vi "ADFGVX.vi"() -> ()   [LabVIEW 2013]
uses:
  <vilib>/Utility/miscctls.llb/LVRowAndColumnTypeDef.ctl
panel:
  out "Intermediate4":string[][](array[string])
  out "Sorted String":string[](array[string])
  out "Intermediate3":string[][](array[string])
  out "Output":string
  out "Intermediate2":string[][](array[string])
  in  "Decrypt":bool
  in  "Encrypt":bool
  in  "Input":string
  out "String1":string caption="Intermediate1"
  in  "String":string
  in  "Stop":bool
  in  "Generate":bool
  in  "Cipher Table":string[][](table)
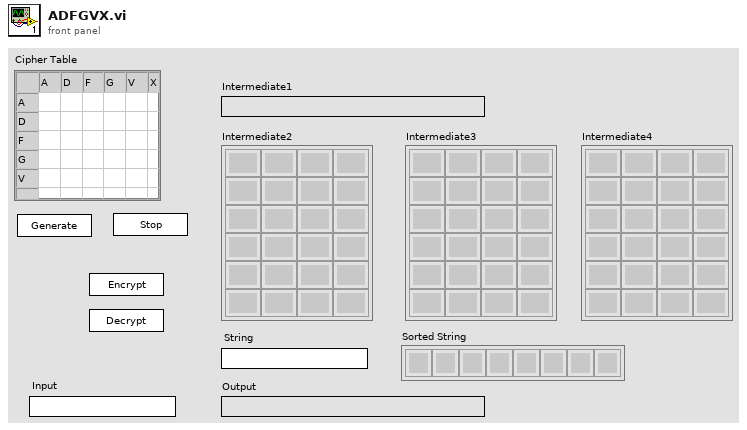
[diagram p1: front panel]
types:
  T1 = typedef "LVRowAndColumnTypeDef.ctl" = cluster{"Row":i32, "Column":i32}
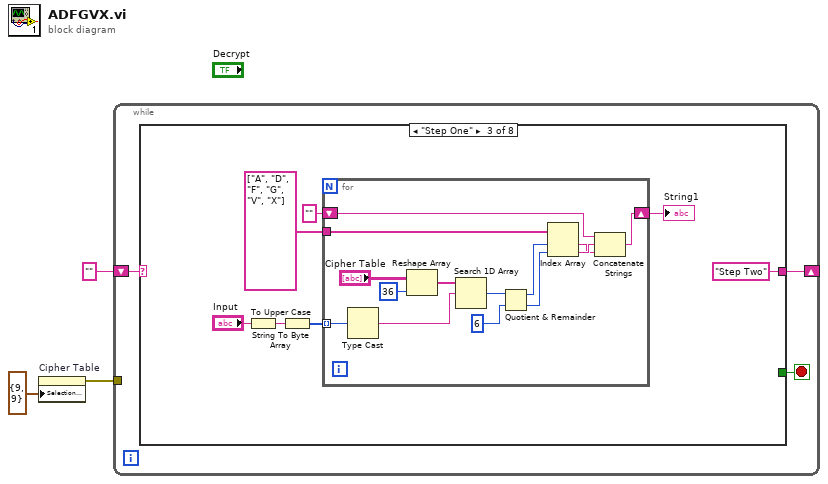
[diagram p0: block diagram]
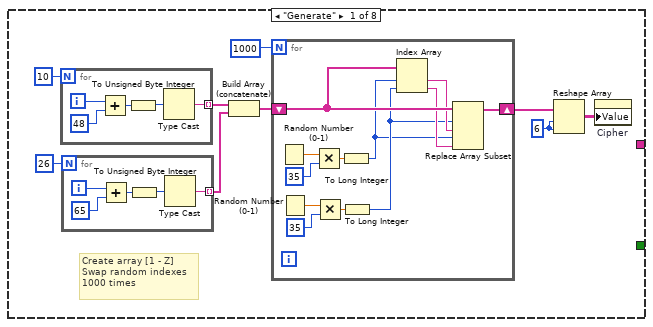
[diagram p2: hidden frame]
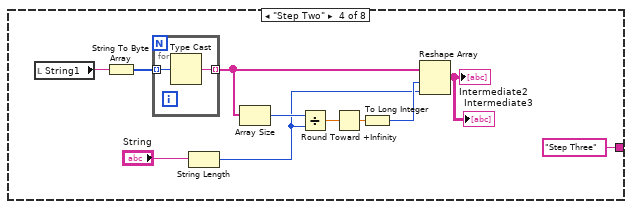
[diagram p4: hidden frame]
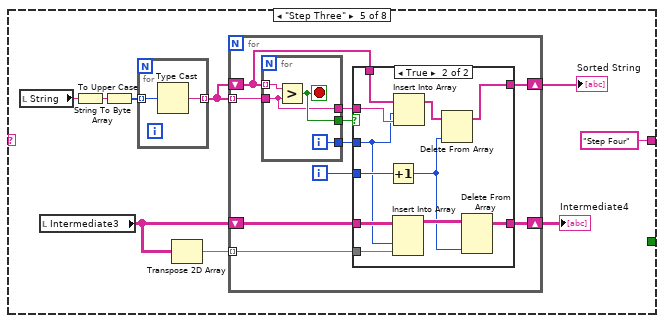
[diagram p5: hidden frame]
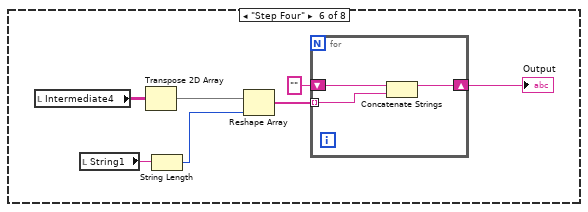
[diagram p7: hidden frame]
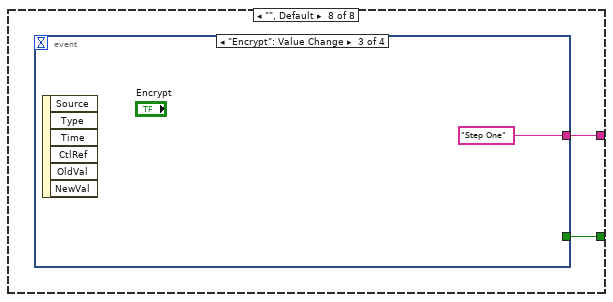
[diagram p9: hidden frame]
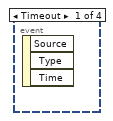
[diagram p10: hidden frame]
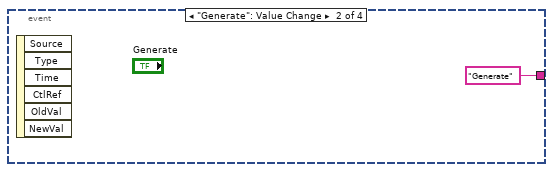
[diagram p11: hidden frame]
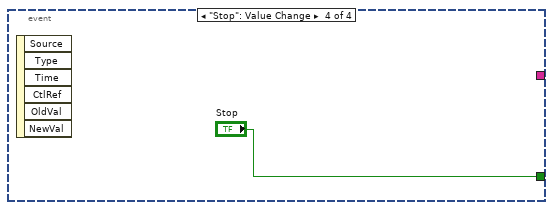
[diagram p12: hidden frame]
diagram:
  n1 = property on="Cipher Table" class="Tbl (strict)"("Selection Start"=T1 {"Row"=9, "Column"=9} ("Active Cell:Active Cell")) -> (error out=w2:errorcluster)  [unwired: 2 in, 1 out]
  n2 = while {
    shift-right: [w5] -> _
    shift-left: "" -> [w6]
    tunnel: w2 -> [_]
    stop <- w4 stop-if-true
    n3 = case shown="\"Step One\"" w6 {
      tunnel: [_ _ "Step Two" "Step Three" "Step Four" _ _ w121] -> w5
      tunnel: [_ _ _ _ _ _ _ w120] -> w4
      frame "Generate" {
        w10 = 6 ("dimension size")
        # "Create array [1 - Z]\nSwap random indexes\n1000 times"
        n4 = for {
          N: 10 -> [_]
          tunnel: [w37] -> w13 mode=indexing
          i -> [w35]
          n5 = Add(x=w35, y=48 ("x")) -> (x+y=w33:i32)
          n6 = To Unsigned Byte Integer(number=w33) -> (unsigned 8bit integer=w36:u8)
          n7 = Type Cast(x=w36) -> (*(type *) &x=w37:string)  [unwired: 1 in]
        }
        n8 = for {
          N: 26 -> [_]
          tunnel: [w32] -> w12 mode=indexing
          i -> [w30]
          n9 = Add(x=w30, y=65 ("x")) -> (x+y=w28:i32)
          n10 = To Unsigned Byte Integer(number=w28) -> (unsigned 8bit integer=w31:u8)
          n11 = Type Cast(x=w31) -> (*(type *) &x=w32:string)  [unwired: 1 in]
        }
        n12 = Build Array (concatenate)(w13, w12) -> (w9:string[])
        n13 = for {
          N: 1000 -> [_]
          shift-right: [w16] -> w7
          shift-left: w9 -> [w24]
          n14 = Random Number (0-1)() -> (number: 0 to 1=w26:dbl)
          n15 = Random Number (0-1)() -> (number: 0 to 1=w22:dbl)
          n16 = Multiply(x=w26, y=35 ("dimension size")) -> (x*y=w27:dbl)
          n17 = Multiply(x=w22, y=35 ("dimension size")) -> (x*y=w21:dbl)
          n18 = To Long Integer(number=w27) -> (32bit integer=w17:i32)
          n19 = To Long Integer(number=w21) -> (32bit integer=w18:i32)
          n20 = Index Array(array=w24, index #1=w17, index #2=w18) -> (element #1=w20:string, element #2=w19:string)
          n21 = Replace Array Subset(array=w24, new element #1=w20, index #1=w18, new element #2=w19, index #2=w17) -> (w16:string[])
        }
        n22 = Reshape Array(w7, w10, w10) -> (w11:string[][])
        n23 = property on="Cipher" class="Tbl (strict)"("Value"=w11) -> ()  [unwired: 2 in, 2 out]
      }
      frame "/** Encrypt **/" {
      }
      frame "Step One" {
        n24 = To Upper Case(1:"Input") -> (0:w41:string)
        n25 = String To Byte Array(string=w41) -> (unsigned byte array=w43:u8[])
        n26 = for {
          tunnel: w43 -> [w58] mode=indexing
          tunnel: string[] ["A", "D", "F", "G", "V", "X"] -> [w51]
          shift-right: [w48] -> w39
          shift-left: "" -> [w47]
          n27 = Type Cast(x=w58) -> (*(type *) &x=w54:string)  [unwired: 1 in]
          n28 = Reshape Array("Cipher Table", 36 ("dimension size")) -> (w55:string[])
          n29 = Search 1D Array(1D array=w55, element=w54) -> (index of element=w53:i32)  [unwired: 1 in]
          n30 = Quotient & Remainder(x=w53, y=6) -> (x-y*floor(x/y)=w49:i32, floor(x/y)=w50:i32)
          n31 = Index Array(array=w51, index #1=w49, index #2=w50) -> (element #1=w45:string, element #2=w46:string)
          n32 = Concatenate Strings(w47, w46, w45) -> (w48:string)
        }
        "String1" <- w39
      }
      frame "Step Two" {
        n33 = local read "String1"() -> (w69:string)
        n34 = String To Byte Array(string=w69) -> (unsigned byte array=w68:u8[])
        n35 = for {
          tunnel: w68 -> [w71] mode=indexing
          tunnel: [w70] -> w66 mode=indexing
          n36 = Type Cast(x=w71) -> (*(type *) &x=w70:string)  [unwired: 1 in]
        }
        n37 = String Length(string="String") -> (length=w61:i32)
        n38 = Array Size(array=w66) -> (size(s)=w65:i32)
        n39 = Divide(x=w65, y=w61) -> (x/y=w64:dbl)
        n40 = Round Toward +Infinity(x=w64) -> (ceil(x): smallest int >= x=w63:dbl)
        n41 = To Long Integer(number=w63) -> (32bit integer=w62:i32)
        n42 = Reshape Array(w66, w62, w61) -> (→"Intermediate2" →"Intermediate3":string[][])
      }
      frame "Step Three" {
        n43 = local read "String"() -> (w79:string)
        n44 = local read "Intermediate3"() -> (w74:string[][])
        n45 = To Upper Case(1:w79) -> (0:w75:string)
        n46 = String To Byte Array(string=w75) -> (unsigned byte array=w78:u8[])
        n47 = for {
          tunnel: w78 -> [w109] mode=indexing
          tunnel: [w108] -> w77 mode=indexing
          n48 = Type Cast(x=w109) -> (*(type *) &x=w108:string)  [unwired: 1 in]
        }
        n49 = Transpose 2D Array(2D array=w74) -> (transposed array=w72:string[][])
        n50 = for {
          tunnel: w77 -> [w90] mode=indexing
          shift-right: [w88] -> w76
          shift-left: w77 -> [w89]
          tunnel: w72 -> [w82] mode=indexing
          shift-right: [w81] -> w73
          shift-left: w74 -> [w83]
          i -> [w84]
          n51 = for {
            tunnel: w90 -> [w104]
            tunnel: w89 -> [w107] mode=indexing
            tunnel: [w106] -> w87
            tunnel: [w105] -> w86
            tunnel: [w104] -> w85
            i -> [w106]
            stop <- w105 stop-if-true
            n52 = Greater?(x=w107, y=w104) -> (0:w105:bool)
          }
          n53 = case shown="True" w86 {
            tunnel: w89 -> [w92 w103]
            tunnel: [w92 w100] -> w88
            tunnel: w87 -> [_ w94]
            tunnel: w85 -> [_ w102]
            tunnel: w84 -> [_ w99]
            tunnel: w83 -> [w91 w98]
            tunnel: w82 -> [_ w97]
            tunnel: [w91 w95] -> w81
            frame False {
            }
            frame True {
              n54 = Increment(x=w99) -> (x+1=w93:i32)
              n55 = Insert Into Array(array=w98, index (col)=w94, new element=w97) -> (w96:string[][])  [unwired: 1 in]
              n56 = Insert Into Array(array=w103, index=w94, new element=w102) -> (w101:string[])
              n57 = Delete From Array(array=w101, index=w93) -> (array with subset deleted=w100:string[])  [unwired: 1 in, 1 out]
              n58 = Delete From Array(array=w96, index (col)=w93) -> (array with subset deleted=w95:string[][])  [unwired: 2 in, 1 out]
            }
          }
        }
        "Sorted String" <- w76
        "Intermediate4" <- w73
      }
      frame "Step Four" {
        n59 = local read "Intermediate4"() -> (w111:string[][])
        n60 = local read "String1"() -> (w116:string)
        n61 = Transpose 2D Array(2D array=w111) -> (transposed array=w110:string[][])
        n62 = String Length(string=w116) -> (length=w115:i32)
        n63 = Reshape Array(w110, w115) -> (w114:string[])
        n64 = for {
          tunnel: w114 -> [w119] mode=indexing
          shift-right: [w118] -> w112
          shift-left: "" -> [w117]
          n65 = Concatenate Strings(w117, w119) -> (w118:string)
        }
        "Output" <- w112
      }
      frame "/** Decrypt **/" {
      }
      frame "", Default {
        n66 = event shown="[2] \"Encrypt\": Value Change" {
          selector: _ -> [_ _ _ _]
          dyn-events: _ -> [_ _ _ _]
          timeout: _ -> [_ _ _ _]
          tunnel: [_ "Generate" "Step One" _] -> w121
          tunnel: [_ _ _ "Stop"] -> w120
          event Timeout {
            n67 = event-data() -> ()  [unwired: 1 in, 3 out]
          }
          event "Generate": Value Change {
            n68 = event-data() -> ()  [unwired: 1 in, 6 out]
          }
          event "Encrypt": Value Change {
            n69 = event-data() -> ()  [unwired: 1 in, 6 out]
          }
          event "Stop": Value Change {
            n70 = event-data() -> ()  [unwired: 1 in, 6 out]
          }
        }
      }
    }
  }
